vi "NDMotor_VISAQuery.vi"() -> ()   [LabVIEW 2024]
panel:
  out "error out":errorcluster
  out "read buffer":string
  in  "write buffer":string
  in  "VISA resource name":refnum<visa-resource-name>
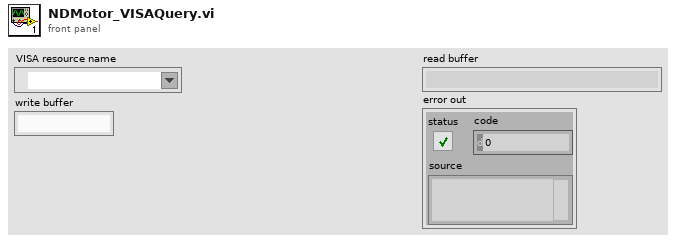
[diagram p1: front panel]
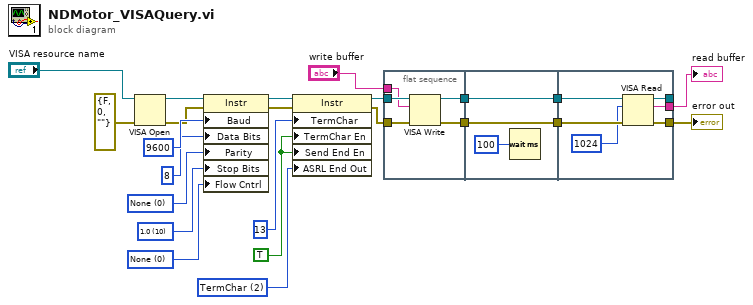
[diagram p0: block diagram]
diagram:
  w14 = u16 0 items=["None", "XON/XOFF", "RTS/CTS", "XON/XOFF & RTS/CTS", "DTR/DSR", "XON/XOFF & DTR/DSR"] ("Serial Settings:Flow Control")
  w15 = u16 10 items=["1.0"=10, "1.5"=15, "2.0"=20] ("Serial Settings:Stop Bits")
  w16 = u16 0 items=["None", "Odd", "Even", "Mark", "Space"] ("Serial Settings:Parity")
  w20 = u16 2 items=["None", "Last Bit", "TermChar", "Break"] ("Serial Settings:End Mode for Writes")
  w22 = TRUE
  n1 = VISA Open(error in (no error)=errorcluster {"status"=FALSE, "code"=0, "source"=""}, VISA resource name="VISA resource name") -> (VISA resource name=w2:refnum<visa-resource-name>, error out=w3:errorcluster)  [unwired: 3 in]
  n2 = property class="Instr"(reference=w2, error in=w3, "Baud"=u32 9600 ("Serial Settings:Baud Rate"), "Data Bits"=u16 8 ("Serial Settings:Data Bits"), "Parity"=w16, "Stop Bits"=w15, "Flow Cntrl"=w14) -> (reference out=w19:refnum<visa-resource-name>, error out=w4:errorcluster)
  n3 = property class="Instr"(reference=w19, error in=w4, "TermChar"=u8 13 ("Termination Character"), "TermChar En"=w22, "Send End En"=w22, "ASRL End Out"=w20) -> (reference out=w12:refnum<visa-resource-name>, error out=w5:errorcluster)
  n4 = flat-sequence {
    tunnel: w12 -> [w28]
    tunnel: [w27] -> w11
    tunnel: [w26] -> w9
    tunnel: "write buffer" -> [w25]
    tunnel: w5 -> [w24]
    tunnel: w11 -> [w31]
    tunnel: [w31] -> w10
    tunnel: w9 -> [w29]
    tunnel: [w29] -> w8
    tunnel: w10 -> [w37]
    tunnel: [w36] -> _
    tunnel: [w35] -> w1
    tunnel: w8 -> [w34]
    tunnel: [w33] -> w6
    frame #0 {
      n5 = VISA Write(VISA resource name=w28, write buffer=w25, error in (no error)=w24) -> (VISA resource name out=w27:refnum<visa-resource-name>, error out=w26:errorcluster)  [unwired: 1 out]
    }
    frame #1 {
      n6 = Wait (ms)(milliseconds to wait=u32 100) -> ()  [unwired: 1 out]
    }
    frame #2 {
      n7 = VISA Read(VISA resource name=w37, byte count=u32 1024, error in (no error)=w34) -> (VISA resource name out=w36:refnum<visa-resource-name>, read buffer=w33:string, error out=w35:errorcluster)  [unwired: 1 out]
    }
  }
  "read buffer" <- w6
  "error out" <- w1
